vi "Register Worker.vi"(8 "error in (no error)":errorcluster, 10 "Worker":refnum<class "Job Handler.lvclass">, 11 "Process Job in":refnum<class "Job Handler.lvclass">) -> (0 "error out":errorcluster, 3 "Process Job out":refnum<class "Job Handler.lvclass">)   [LabVIEW 2020, in "Job Handler.lvclass"]
uses:
  Job Handler.lvclass
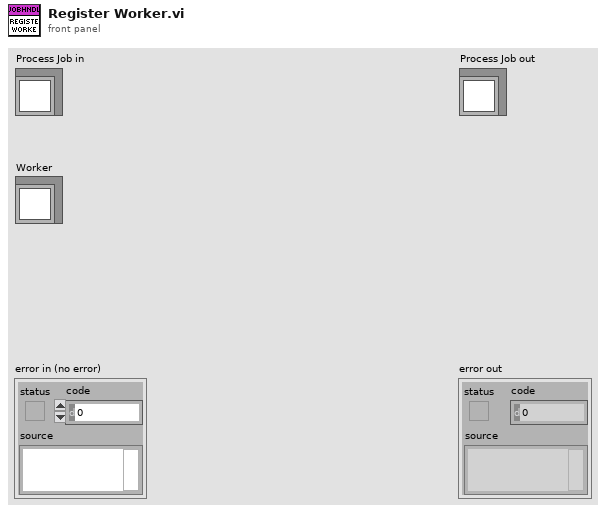
[diagram p1: front panel]
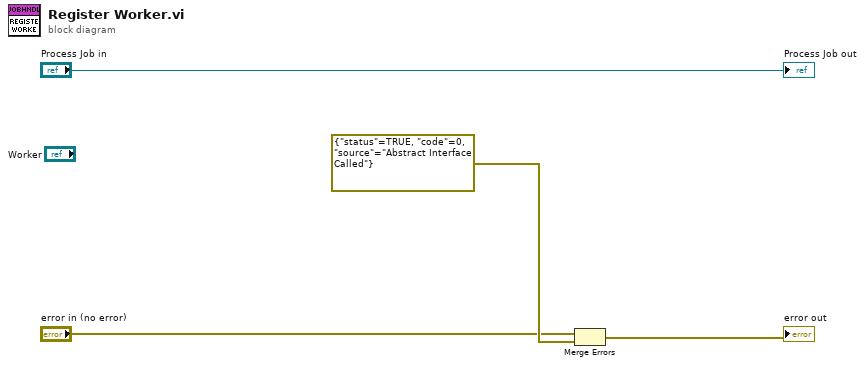
[diagram p0: block diagram]
diagram:
  n1 = Merge Errors("error in (no error)", errorcluster {"status"=TRUE, "code"=0, "source"="Abstract Interface Called"} ("error in (no error)")) -> (→"error out":errorcluster)
  "Process Job out" <- "Process Job in"
